vi "GetWidthHeight.vi"(0 "reference in":refnum<class "Map.lvclass">, 5 "error in (no error)":errorcluster) -> (14 "reference out":refnum<class "Map.lvclass">, 15 "Width":i32, 16 "Height":i32, 19 "error out":errorcluster)   [LabVIEW 2020, in "Map.lvclass"]
doc: "Get size of Map"
uses:
  Map.lvclass
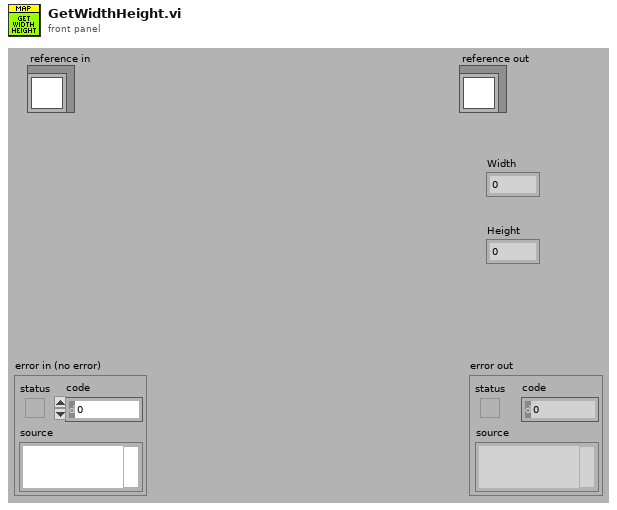
[diagram p1: front panel]
types:
  T1 = typedef "Map.lvclass/ObjectAttributes.ctl" = cluster{"Width":i32, "Height":i32, "Map":bool[][]}
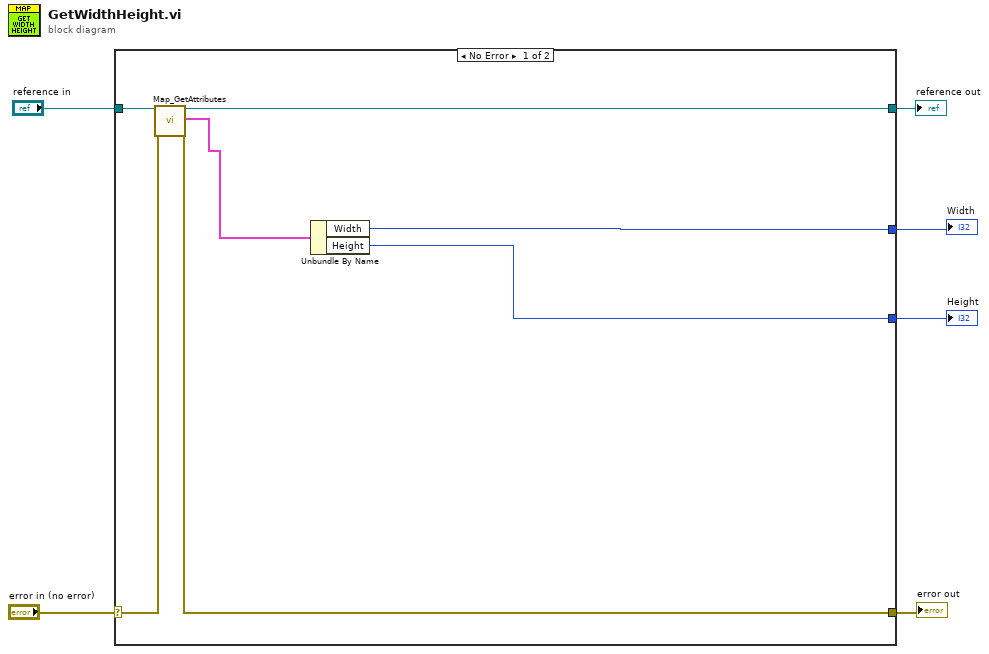
[diagram p0: block diagram]
diagram:
  n1 = case shown="No Error" "error in (no error)" {
    selector: "error in (no error)" -> [w13 w15]
    tunnel: [w12 w15] -> w5
    tunnel: [w10 w14] -> w3
    tunnel: "reference in" -> [w11 w14]
    tunnel: [w8 _] -> w2
    tunnel: [w7 _] -> w1
    frame No Error {
      n2 = call "Map_GetAttributes.vi"("reference in"=w11, "error in (no error)"=w13) -> ("reference out"=w10:refnum<class "Map.lvclass">, "Attributes"=w9:T1, "error out"=w12:errorcluster)  [unwired: 15 out]
      n3 = Unbundle By Name(w9) -> ("Width"=w8:i32, "Height"=w7:i32)
    }
    frame Error {
    }
  }
  "error out" <- w5
  "reference out" <- w3
  "Width" <- w2
  "Height" <- w1
